vi "FilterWaveformData.vi"(8 "error in (no error)":errorcluster, 10 "923x Acquisition Config":T1 {"HighPassFilterState"."Filter State" format="%.2f"; "HighPassFilterState"."IIR Filter Cluster"."Forward Coefficients" format="%.2f"; "HighPassFilterState"."IIR Filter Cluster"."Reverse Coefficients" format="%.2f"; "FixedSizeX32"."InputConfig" items=["AC Coupled", "DC Coupled", "IEPE AC Coupled"]}, 11 "waveforms in":waveform(sgl)[](array[waveform])) -> (0 "error out":errorcluster, 2 "923x Acquisition Config out":T1 {"HighPassFilterState"."Filter State" format="%.2f"; "HighPassFilterState"."IIR Filter Cluster"."Forward Coefficients" format="%.2f"; "HighPassFilterState"."IIR Filter Cluster"."Reverse Coefficients" format="%.2f"; "FixedSizeX32"."InputConfig" items=["AC Coupled", "DC Coupled", "IEPE AC Coupled"]}, 3 "waveforms out":waveform(sgl)[](array[waveform]))   [LabVIEW 2017, in "CmsAcquisition.lvlib"]
uses:
  <vilib>/addons/InsightCM/Devices/Shared/Cms/CmsAcquisition/CmsAcquisition.lvlib
  <vilib>/addons/InsightCM/Devices/Shared/Cms/CmsAcquisition/controls/Configuration.ctl
  <vilib>/addons/InsightCM/Devices/Shared/Cms/CmsAcquisition/controls/TachometerConfig.ctl
  <vilib>/addons/InsightCM/Devices/Shared/Cms/CmsAcquisition/controls/FixedSizeArrays.ctl
  <vilib>/LabVIEW Targets/FPGA/cRIO/shared/nicrio_ModuleControls/nicrio_cRIO-9232_ConfigModeRing.ctl
  <vilib>/addons/InsightCM/Devices/Shared/Cms/cRIOWfmAcq/subVIs/RIO Wfm Cust Ctrls/rwfm_SamplingInfo.ctl
  <vilib>/addons/InsightCM/Devices/Shared/Cms/CmsAcquisition/controls/Group.ctl
  <vilib>/addons/InsightCM/Devices/Shared/Cms/CmsAcquisition/controls/Channel.ctl
  <vilib>/addons/InsightCM/Utilities/Analysis/Vibration/controls/HighPassFilterState.ctl
  <vilib>/addons/InsightCM/Devices/Shared/Cms/CmsAcquisition/controls/BurstMode.ctl
  <vilib>/addons/InsightCM/Utilities/Analysis/Vibration/VibrationAnalysisFunctions.lvlib
  <vilib>/addons/InsightCM/Devices/Shared/Cms/cRIOWfmAcq/cRIOWfmLib.lvlib
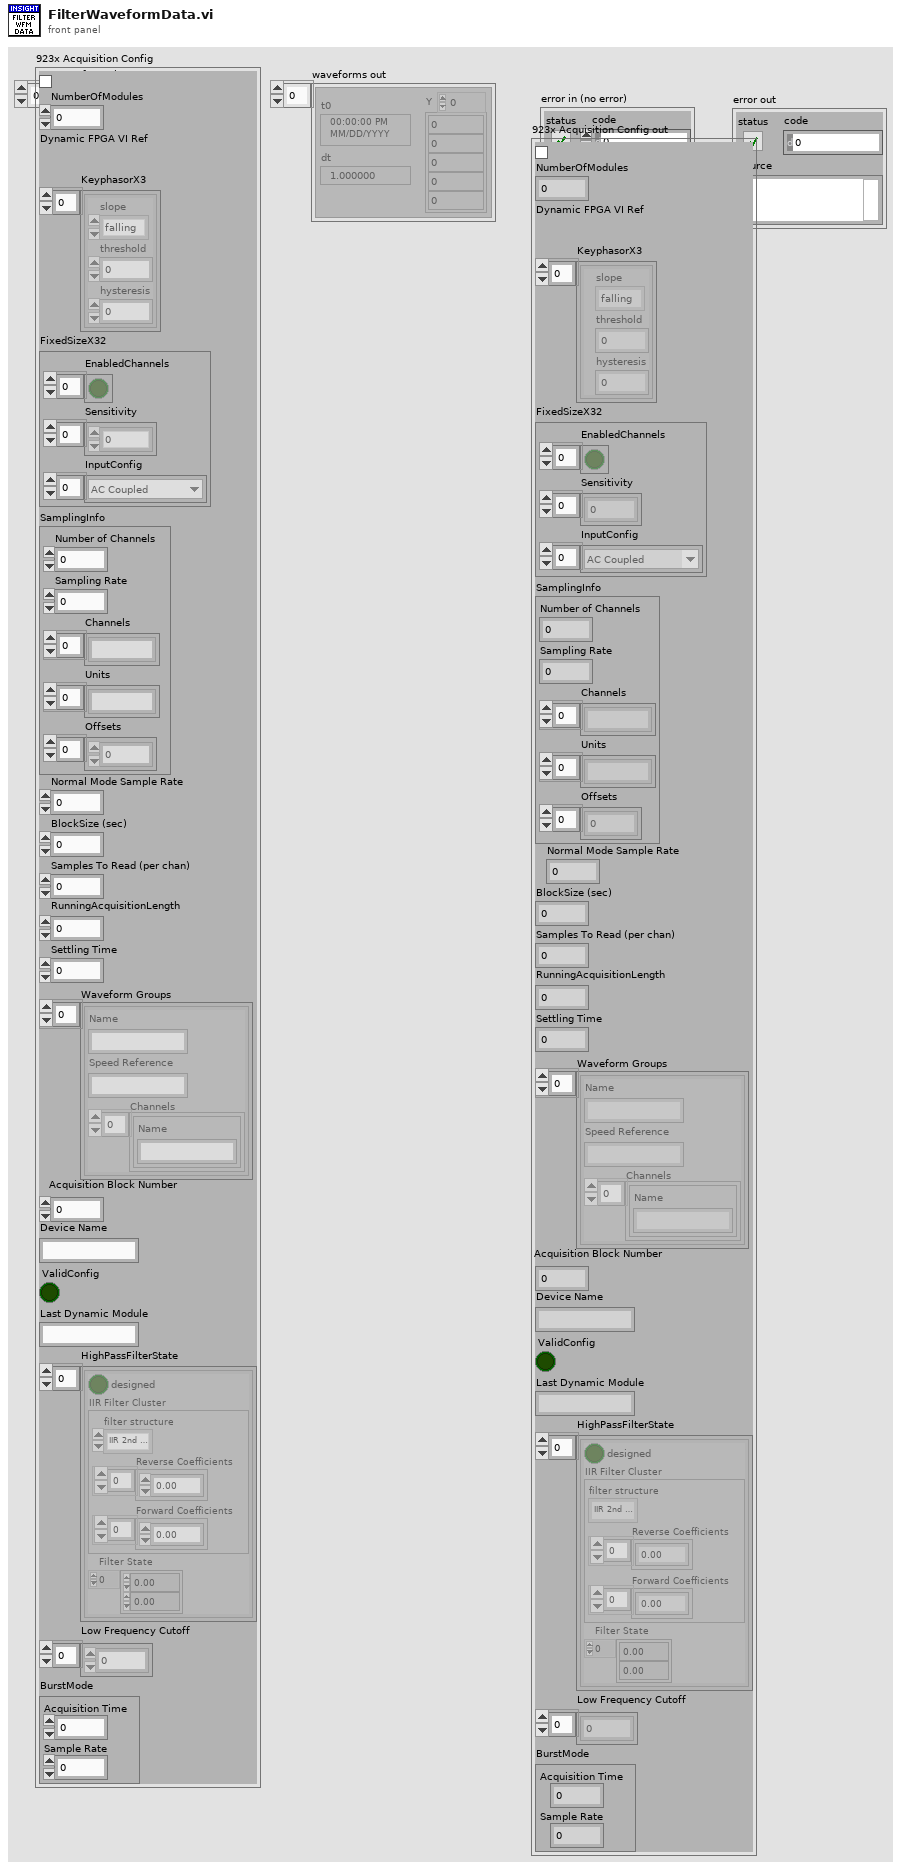
[diagram p1: front panel]
types:
  T1 = typedef "CmsAcquisition.lvlib/Configuration.ctl" = cluster{"Acq":bool, "NumberOfModules":i16, "Dynamic FPGA VI Ref":refnum<k20>, "KeyphasorX3":T2[], "FixedSizeX32":T3, "SamplingInfo":T5, "Normal Mode Sample Rate":dbl, "BlockSize (sec)":dbl, "Samples To Read (per chan)":i32, "RunningAcquisitionLength":dbl, "Settling Time":dbl, "Waveform Groups":T6[], "Acquisition Block Number":i32, "Device Name":string, "ValidConfig":bool, "Last Dynamic Module":string, "HighPassFilterState":T8[], "Low Frequency Cutoff":dbl[], "BurstMode":T9}
  T2 = typedef "CmsAcquisition.lvlib/TachometerConfig.ctl" = cluster{"slope":enum16{"falling", "rising"}, "threshold":dbl, "hysteresis":dbl}
  T3 = typedef "CmsAcquisition.lvlib/FixedSizeArrays.ctl" = cluster{"EnabledChannels":bool[], "Sensitivity":dbl[], "InputConfig":T4[]}
  T4 = typedef "nicrio_cRIO-9232_ConfigModeRing.ctl" = u8
  T5 = typedef "cRIOWfmLib.lvlib/rwfm_SamplingInfo.ctl" = cluster{"Number of Channels":i32, "Sampling Rate":dbl, "Channels":string[], "Units":string[], "Offsets":sgl[]}
  T6 = typedef "CmsAcquisition.lvlib/Group.ctl" = cluster{"Name":string, "Speed Reference":string, "Channels":T7[]}
  T7 = typedef "CmsAcquisition.lvlib/Channel.ctl" = cluster{"Name":string}
  T8 = typedef "VibrationAnalysisFunctions.lvlib/HighPassFilterState.ctl" = cluster{"designed":bool, "IIR Filter Cluster":cluster{"filter structure":enum32{"IIR 2nd Order", "IIR 4th Order"}, "Reverse Coefficients":dbl[], "Forward Coefficients":dbl[]}, "Filter State":dbl[]}
  T9 = typedef "CmsAcquisition.lvlib/BurstMode.ctl" = cluster{"Acquisition Time":dbl, "Sample Rate":dbl}
  T10 = cluster{"filter structure":enum32{"IIR 2nd Order", "IIR 4th Order"}, "Reverse Coefficients":dbl[], "Forward Coefficients":dbl[]}
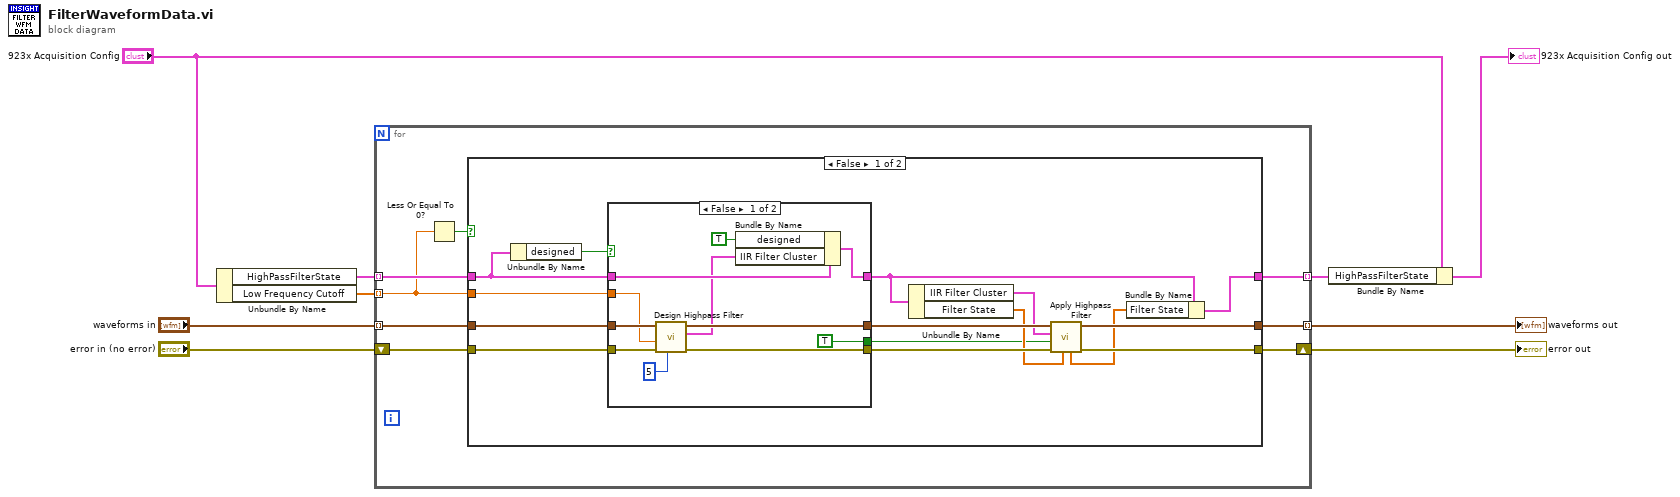
[diagram p0: block diagram]
diagram:
  n1 = Unbundle By Name("923x Acquisition Config") -> ("HighPassFilterState"=w5:T8[], "Low Frequency Cutoff"=w1:dbl[])
  n2 = for {
    tunnel: "waveforms in" -> [w17] mode=indexing
    tunnel: [w15] -> w7 mode=indexing
    shift-right: [w14] -> w6
    shift-left: "error in (no error)" -> [w16]
    tunnel: w5 -> [w13] mode=indexing
    tunnel: [w12] -> w2 mode=indexing
    tunnel: w1 -> [w10] mode=indexing
    n3 = Less Or Equal To 0?(x=w10) -> (x <= 0?=w11:bool)
    n4 = case shown="False" w11 {
      tunnel: w17 -> [w32 w48]
      tunnel: w16 -> [w31 w47]
      tunnel: [w28 w48] -> w15
      tunnel: [w27 w47] -> w14
      tunnel: w10 -> [w25 _]
      tunnel: w13 -> [w24 w49]
      tunnel: [w18 w49] -> w12
      frame False {
        n5 = Unbundle By Name(w24) -> ("designed"=w26:bool)
        n6 = case shown="False" w26 {
          tunnel: w32 -> [w43 w46]
          tunnel: w31 -> [w42 w45]
          tunnel: [w41 w46] -> w30
          tunnel: [w40 w45] -> w29
          tunnel: w25 -> [w38 _]
          tunnel: w24 -> [w37 w44]
          tunnel: [w34 w44] -> w20
          tunnel: [TRUE ("init/cont (init:F)") _] -> w21
          frame False {
            n7 = call <vilib>:"Design Highpass Filter.vi"("highpass filter order"=5, "error in (no error)"=w42, "highpass cutoff frequency"=w38, "input signal"=w43) -> ("error out"=w40:errorcluster, "IIR Filter Cluster"=w36:T10, "dup signal"=w41:waveform(sgl))  [unwired: 5 in]
            n8 = Bundle By Name(cluster=w37, "designed"=TRUE, "IIR Filter Cluster"=w36) -> (w34:T8)
          }
          frame True {
          }
        }
        n9 = Unbundle By Name(w20) -> ("IIR Filter Cluster"=w23:T10, "Filter State"=w22:dbl[])
        n10 = call <vilib>:"Apply Highpass Filter.vi"("Initial Filter State"=w22, "error in (no error)"=w29, "init/cont (init:F)"=w21, "filter coefficients"=w23, "signal [V]"=w30) -> ("error out"=w27:errorcluster, "filtered signal [EU]"=w28:waveform(sgl), "Final Filter State"=w19:dbl[])  [unwired: 4 in]
        n11 = Bundle By Name(cluster=w20, "Filter State"=w19) -> (w18:T8)
      }
      frame True {
      }
    }
  }
  "waveforms out" <- w7
  "error out" <- w6
  n12 = Bundle By Name(cluster="923x Acquisition Config", "HighPassFilterState"=w2) -> (→"923x Acquisition Config out":T1)
